vi "test scratch.vi"() -> ()   [LabVIEW 2013]
panel:
  in  "x":i32
  out "Array":string[](array[string])
  in  "Stop Button":bool
  out "decimal integer string":string
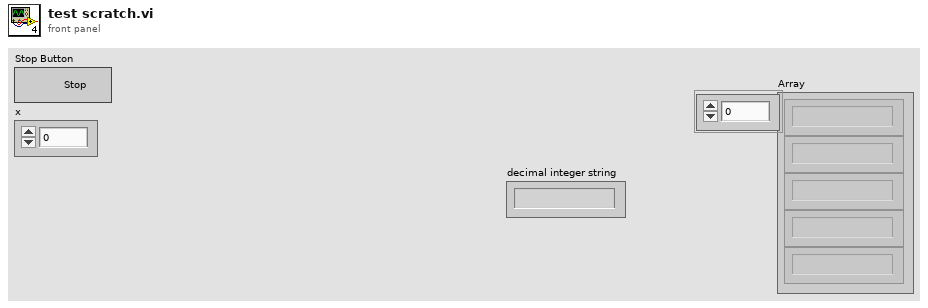
[diagram p1: front panel]
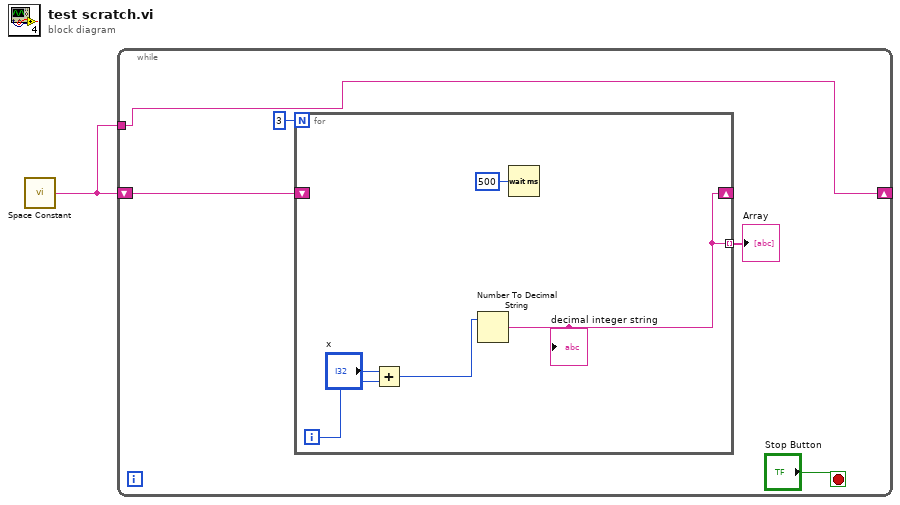
[diagram p0: block diagram]
diagram:
  n1 = call <vilib>:"Space Constant.vi"() -> ("String"=w1:string)
  n2 = while {
    shift-right: [w5] -> _
    shift-left: w1 -> [w6]
    tunnel: w1 -> [w5]
    stop <- "Stop Button" stop-if-true
    n3 = for {
      N: 3 -> [_]
      shift-right: [w11] -> _
      shift-left: w6 -> [_]
      tunnel: [w11] -> w2 mode=indexing
      i -> [w9]
      n4 = Add(x="x", y=w9) -> (x+y=w8:i32)
      n5 = Number To Decimal String(number=w8) -> (decimal integer string=w11:string)  [unwired: 1 in]
      "decimal integer string" <- w11
      n6 = Wait (ms)(milliseconds to wait=u32 500) -> ()  [unwired: 1 out]
    }
    "Array" <- w2
  }
